vi "Create VariantBufferMap.vi"(8 "error in":errorcluster, 11 "bufSize":i32) -> (0 "error out":errorcluster, 3 "BufferMap":refnum<data-value>)   [LabVIEW 2013, in "VariantBufferMap.lvclass"]
doc: "This VI creates a ring buffer of set size. This buffer is created in one place in the memory and is then accessed via pointer/reference.\n\nThe Data Type input is required because it defines the place in the memory to correct size thus removing the need for memory reallocation."
uses:
  VariantBufferMap.lvclass
  VariantBufferMap.lvclass/VariantBufferMap.ctl
  VariantBuffer/VariantBuffer.lvclass
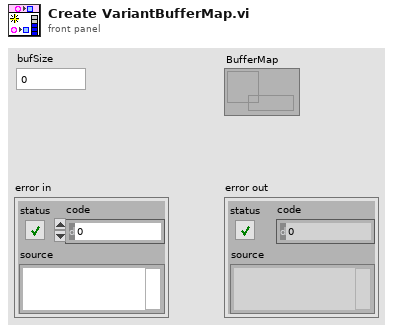
[diagram p1: front panel]
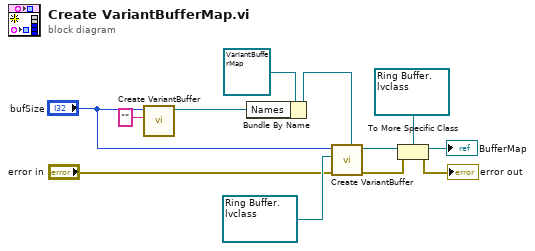
[diagram p0: block diagram]
diagram:
  n1 = call "Create VariantBuffer.vi"("default"="", "bufSize"="bufSize") -> ("Buffer"=w8:refnum<data-value>)  [unwired: 8 in, 1 out]
  n2 = Bundle By Name(cluster=refnum<class "VariantBufferMap.lvclass"> refnum ("Ring Buffer.lvclass"), "Names"=w8) -> (w7:refnum<class "VariantBufferMap.lvclass">)
  n3 = call "Create VariantBuffer.vi"("Buffer"=w7, "error in"="error in", "default"=refnum<data-value> refnum ("Buffer"), "bufSize"="bufSize") -> ("error out"=w1:errorcluster, "Buffer"=w5:refnum<data-value>)  [unwired: 6 in]
  n4 = To More Specific Class(target class=refnum<data-value> refnum ("BufferMap"), reference=w5, error in=w1) -> (specific class reference=→"BufferMap":refnum<data-value>, error out=→"error out":errorcluster)
